vi "Saved ARINC Global Items.vi"() -> ()   [LabVIEW 2011]
panel:
  in  "2010MainTemp":string="961BA415-D612-25DB-1EE4-93AC9399C9BC"
  in  "Status Section":string="Status"
  in  "Type":string="Type"
  in  "Label":string="Label"
  in  "txRate":string="txRate"
  in  "transferPeriod":string="transferPeriod"
  in  "Label Section Page GUID":string="961BA415-D612-25DB-1EE4-93AC9399C911"
  in  "Label Data Page GUID":string="961BA415-D612-25DB-1EE4-93AC9399C951"
  in  "Channel Page GUID":string="7E8619EB-70E6-9299-14EE-99E8B20A7109"
  in  "HWOutputs GUID":string="B316C0B3-A1A3-75D9-9053-C890A1BD32E0"
  in  "HWInputs GUID":string="3FB60206-0B92-B78E-8988-3E4A690C747C"
  in  "InBufferSize":string="InBufferSize"
  in  "Channel #":string="Channel #"
  in  "RT File Path":string="RT File Path"
  in  "Outputs":string="Outputs"
  in  "Inputs":string="Inputs"
  in  "WinBinCache":string="Temp429BinFiles"
  in  "ScheduledSDI":string="ScheduledSDI"
  in  "xmlName":string="xmlName"
  in  "SDIValue":string="SDIValue"
  in  "SDI_Enabled":string="SDI_Enabled"
  in  "InputsReadRate":string="InputsReadRate"
  in  "InLoopTime":string="Inputs Loop Duration"
  in  "OutLoopTime":string="Outputs Loop Duration"
  in  "Error Code":string="Error Code"
  in  "HWOut Late Count":string="Outputs Late Count"
  in  "HWIn Late Count":string="Inputs Late Count"
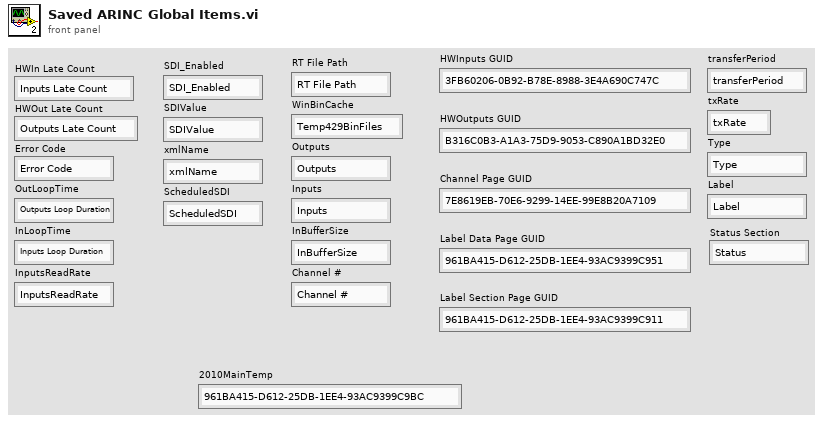
[diagram p1: front panel]
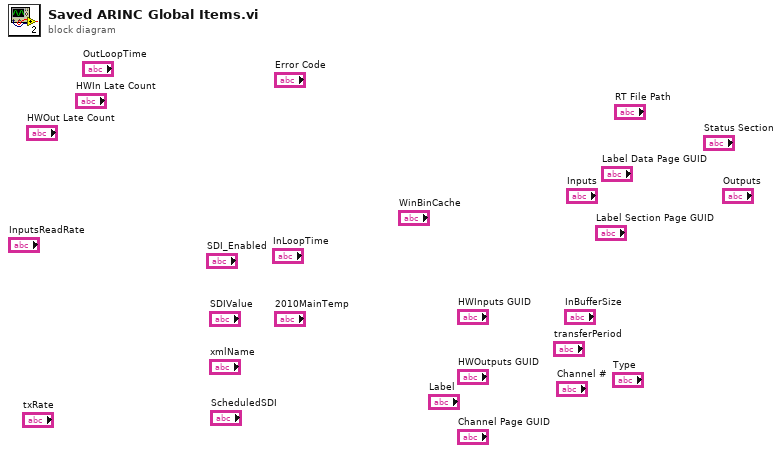
[diagram p0: block diagram]
diagram:
